vi "GetFeatureUnit.vi"(5 "metric":T1, 7 "channel":T3, 8 "error in (no error)":errorcluster, 10 "metric definitionInstance id":string, 11 "metric cache in":variant) -> (0 "error out":errorcluster, 1 "use volts":bool, 2 "unit":string, 3 "metric cache out":variant)   [LabVIEW 2017, in "AnalysisHelper.lvlib"]
uses:
  <vilib>/addons/InsightCM/Utilities/Analysis/Shared/AnalysisHelper.lvlib
  <vilib>/addons/InsightCM/MessageBus/Base/controls/R2_Channel.ctl
  <vilib>/addons/InsightCM/MessageBus/Base/controls/KeyValuePair.ctl
  <vilib>/addons/InsightCM/MessageBus/Base/controls/Metric.ctl
  <vilib>/addons/InsightCM/Utilities/PropertyHelpers/PropertyHelpers.lvlib
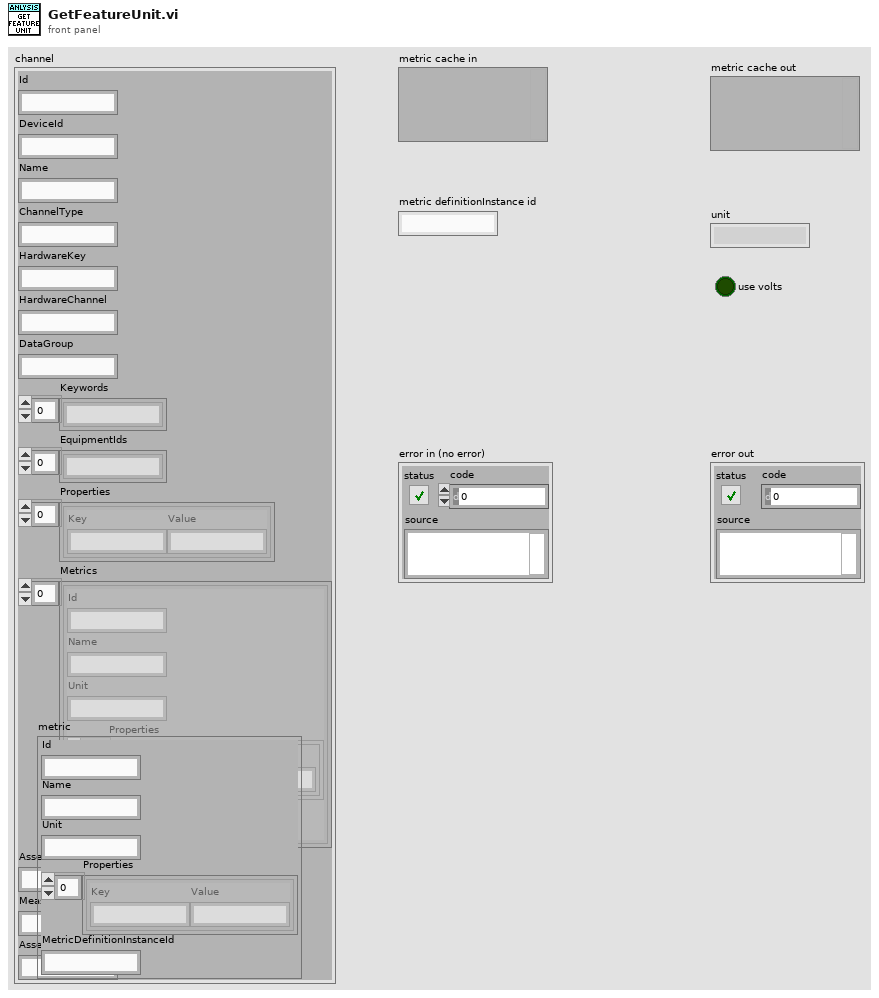
[diagram p1: front panel]
types:
  T1 = typedef "Metric.ctl" = cluster{"Id":string, "Name":string, "Unit":string, "Properties":T2[], "MetricDefinitionInstanceId":string}
  T2 = typedef "KeyValuePair.ctl" = cluster{"Key":string, "Value":string}
  T3 = typedef "R2_Channel.ctl" = cluster{"Id":string, "DeviceId":string, "Name":string, "ChannelType":string, "HardwareKey":string, "HardwareChannel":string, "DataGroup":string, "Keywords":string[], "EquipmentIds":string[], "Properties":T2[], "Metrics":T1[], "AssetNodeId":string, "MeasType":string, "AssetName":string}
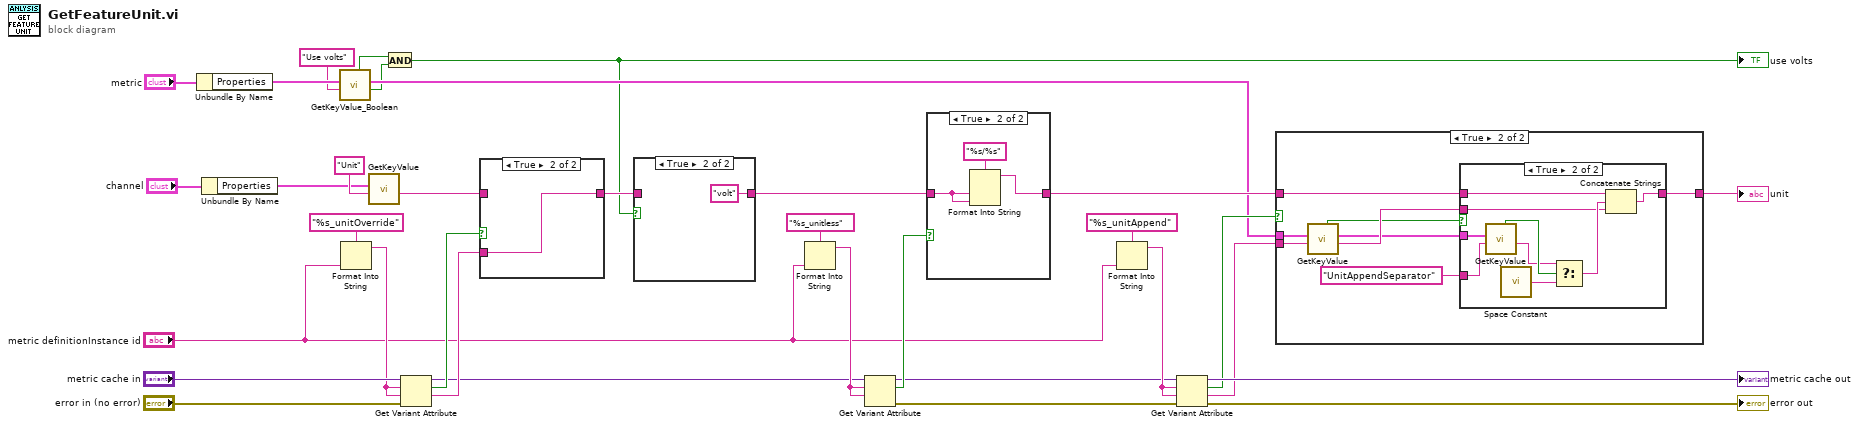
[diagram p0: block diagram]
diagram:
  n1 = Unbundle By Name("metric") -> ("Properties"=w8:T2[])
  n2 = Unbundle By Name("channel") -> ("Properties"=w21:T2[])
  n3 = call <vilib>:"GetKeyValue_Boolean.vi"("key"="Use volts", "key value pairs"=w8) -> ("value"=w4:bool, "key value pairs out"=w7:T2[], "found"=w5:bool)  [unwired: 7 in]
  n4 = Format Into String(format string="%s_unitOverride", "metric definitionInstance id") -> (resulting string=w30:string)  [unwired: 2 in, 1 out]
  n5 = call <vilib>:"GetKeyValue.vi"("key"="Unit" ("name"), "key value pairs"=w21) -> ("value"=w27:string)  [unwired: 7 in, 2 out]
  n6 = And(x=w5, y=w4) -> (x .and. y?=w1:bool)
  "use volts" <- w1
  n7 = Get Variant Attribute(Variant="metric cache in", name=w30, default value (empty Variant)=w30, error in="error in (no error)") -> (duplicate Variant=w23:variant, found=w29:bool, value=w28:string)  [unwired: 1 out]
  n8 = case shown="True" w29 {
    tunnel: [w35 w36] -> w2
    tunnel: w28 -> [_ w36]
    tunnel: w27 -> [w35 _]
    frame False {
    }
    frame True {
    }
  }
  n9 = case shown="True" w1 {
    tunnel: [w37 "volt" ("value")] -> w3
    tunnel: w2 -> [w37 _]
    frame False {
    }
    frame True {
    }
  }
  n10 = Format Into String(format string="%s_unitless", "metric definitionInstance id") -> (resulting string=w26:string)  [unwired: 2 in, 1 out]
  n11 = Get Variant Attribute(Variant=w23, name=w26, default value (empty Variant)=w26) -> (duplicate Variant=w17:variant, found=w24:bool, error out=w14:errorcluster)  [unwired: 1 in, 1 out]
  n12 = case shown="True" w24 {
    tunnel: [w39 w41] -> w10
    tunnel: w3 -> [w39 w40]
    frame False {
    }
    frame True {
      n13 = Format Into String(format string="%s/%s", w40, w40) -> (resulting string=w41:string)  [unwired: 2 in, 1 out]
    }
  }
  n14 = Format Into String(format string="%s_unitAppend", "metric definitionInstance id") -> (resulting string=w19:string)  [unwired: 2 in, 1 out]
  n15 = Get Variant Attribute(Variant=w17, name=w19, default value (empty Variant)=w19, error in=w14) -> (duplicate Variant=→"metric cache out":variant, found=w12:bool, value=w11:string, error out=→"error out":errorcluster)
  n16 = case shown="True" w12 {
    tunnel: w11 -> [_ w48]
    tunnel: w10 -> [w43 w51]
    tunnel: [w43 w50] -> w9
    tunnel: w7 -> [_ w49]
    frame False {
      # "Unit done"
    }
    frame True {
      # "Append a unit"
      n17 = call <vilib>:"GetKeyValue.vi"("key"=w48, "key value pairs"=w49) -> ("value"=w47:string, "key value pairs out"=w45:T2[], "found"=w46:bool)  [unwired: 7 in]
      n18 = case shown="True" w46 {
        tunnel: w45 -> [_ w56]
        tunnel: w51 -> [w52 w60]
        tunnel: w47 -> [_ w58]
        tunnel: [w52 w57] -> w50
        tunnel: "UnitAppendSeparator" ("Key") -> [_ w53]
        frame False {
        }
        frame True {
          n19 = call <vilib>:"GetKeyValue.vi"("key"=w53, "key value pairs"=w56) -> ("value"=w54:string, "found"=w55:bool)  [unwired: 7 in, 1 out]
          n20 = call <vilib>:"Space Constant.vi"() -> ("String"=w61:string)
          n21 = Select(t=w54, s=w55, f=w61) -> (s? t:f=w59:string)
          n22 = Concatenate Strings(w60, w59, w58) -> (w57:string)
        }
      }
    }
  }
  "unit" <- w9
